vi "Excel_File_Open.vi"(1 "File Path and Name":path) -> ()   [LabVIEW 2020]
doc: "This VI illustrates how to print a spreadsheet file using Excel without actually opening\nthe application itself. By using the ActiveX VIs this VI runs the entire print process in\nthe background.\n\nJust enter the full pathname of your spreadsheet file in the Filename string control box\nand run the VI. Your file will then be printed to your default Windows printer. Bear in\nmind that the file must be either an Excel file or an ASCII file in spreadsheet format.\n(The columns are separated by tabs or commas etc.)"
panel:
  in  "Excel._Application":refnum<k7>
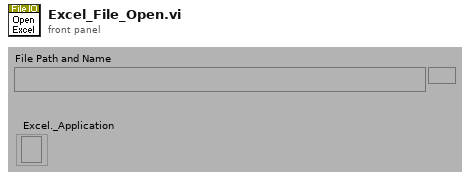
[diagram p1: front panel]
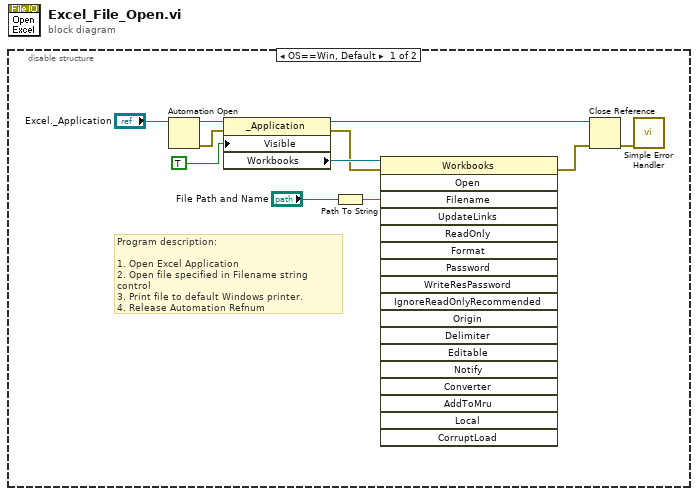
[diagram p0: block diagram]
diagram:
  n1 = disable-structure shown="OS==Win, Default" {
    frame condition #0 (active) {
      # "Program description:\n\n1. Open Excel Application\n2. Open file specified in Filename string control\n3. Print file to default Windows printer.\n4. Release Automation Refnum"
      n2 = Automation Open(Automation Refnum="Excel._Application") -> (Automation Refnum=w11:refnum<k7>, error out=w10:errorcluster)  [unwired: 3 in]
      n3 = property class="_Application"(reference=w11, error in=w10, "Visible"=TRUE) -> (reference out=w3:refnum<k7>, error out=w6:errorcluster, "Workbooks"=w8:refnum<k7>)
      n4 = Path To String(path="File Path and Name") -> (string=w1:string)
      n5 = invoke class="Workbooks" method="Open"(reference=w8, error in=w6, "Filename"=w1) -> (error out=w2:errorcluster)  [unwired: 15 in, 17 out]
      n6 = Close Reference(reference=w3, error in (no error)=w2) -> (error out=w5:errorcluster)
      n7 = call <vilib>:"Simple Error Handler.vi"("error in (no error)"=w5) -> ()  [unwired: 4 in, 5 out]
    }
    frame condition #1 {
    }
  }
